vi "channel to string.vi"(11 "channel in":refnum<class "TBM channel.lvclass">) -> (2 "channel data":string, 3 "identifier":string)   [LabVIEW 2013, in "TBM channel.lvclass"]
doc: "serializes channel.lvclass into an identifier and associated data."
uses:
  TBM channel.lvclass
  <vilib>/NI/Tag Bus/tag/tag descriptor.lvclass/tag descriptor.ctl
  TBM channel.lvclass/TBM channel.ctl
  <vilib>/NI/Tag Bus/tag/tag descriptor.lvclass
  root configuration/TBM configuration.lvclass
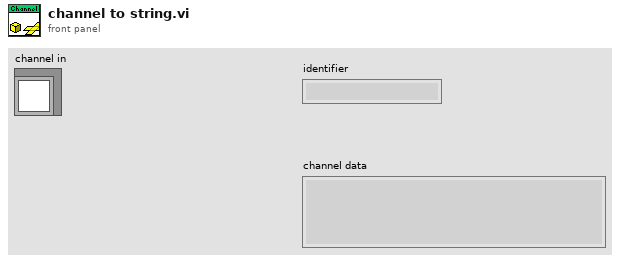
[diagram p1: front panel]
types:
  T1 = typedef "tag bus.lvlib/tag descriptor.lvclass/Data Type.ctl" = enum16{"Double", "Single", "I64", "I32", "I16", "I8", "U64", "U32", "U16", "U8", "Boolean", "String", "Array of Double", "Array of Single", "Array of I64", "Array of I32", "Array of I16", "Array of I8", "Array of U64", "Array of U32", "Array of U16", "Array of U8", "Array of Boolean", "Array of String"}
  T2 = typedef "TBM channel.lvclass/channel classification.ctl" = enum16{"input data", "output data", "processing parameter", "processing result"}
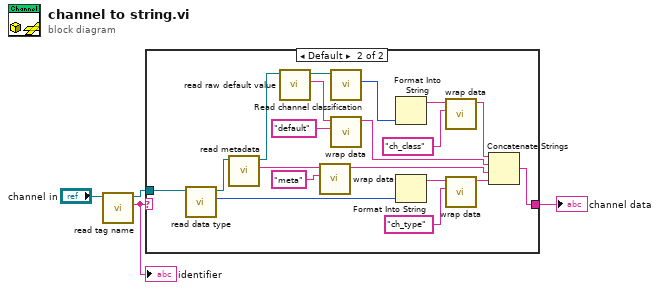
[diagram p0: block diagram]
diagram:
  n1 = call <vilib>:"read tag name.vi"("system tag in"="channel in") -> ("name"=w1:string, "system tag out"=w2:refnum<class "TBM channel.lvclass">)  [unwired: 8 in, 1 out]
  "identifier" <- w1
  n2 = case shown="Default" w1 {
    selector: w1 -> [w5 _]
    tunnel: [w5 w6] -> w4
    tunnel: w2 -> [_ w7]
    frame "" {
    }
    frame Default {
      n3 = call <vilib>:"read data type.vi"("system tag in"=w7) -> ("data type"=w22:T1, "system tag out"=w24:refnum<class "TBM channel.lvclass">)  [unwired: 8 in, 1 out]
      n4 = call <vilib>:"read metadata.vi"("system tag in"=w24) -> ("metadata"=w17:string, "system tag out"=w23:refnum<class "TBM channel.lvclass">)  [unwired: 8 in, 1 out]
      n5 = call <vilib>:"read raw default value.vi"("system tag in"=w23) -> ("raw default"=w16:string, "system tag out"=w19:refnum<class "TBM channel.lvclass">)  [unwired: 8 in, 1 out]
      n6 = call "wrap data.vi"("identifier"="meta", "data to wrap"=w17) -> ("wrapped data"=w9:string)  [unwired: 9 in]
      n7 = call "Read channel classification.vi"("channel in"=w19) -> ("channel classification"=w14:T2)  [unwired: 8 in, 2 out]
      n8 = call "wrap data.vi"("identifier"="default", "data to wrap"=w16) -> ("wrapped data"=w10:string)  [unwired: 9 in]
      n9 = Format Into String(w14) -> (resulting string=w13:string)  [unwired: 3 in, 1 out]
      n10 = Format Into String(w22) -> (resulting string=w21:string)  [unwired: 3 in, 1 out]
      n11 = call "wrap data.vi"("identifier"="ch_class", "data to wrap"=w13) -> ("wrapped data"=w11:string)  [unwired: 9 in]
      n12 = call "wrap data.vi"("identifier"="ch_type", "data to wrap"=w21) -> ("wrapped data"=w8:string)  [unwired: 9 in]
      n13 = Concatenate Strings(w11, w10, w9, w8) -> (w6:string)
    }
  }
  "channel data" <- w4
